vi "LVOOP Custom Probes.vi"() -> ()   [LabVIEW 2020]
doc: "This example demonstrates custom probes with LabVIEW classes.\n\nRefer to the LabVIEW Help for more information about LabVIEW object-oriented programming."
uses:
  Vehicle/Vehicle.lvclass
  Truck/Truck.lvclass
panel:
  out "truck":refnum<class "Truck.lvclass">
  out "vehicle":refnum<class "Vehicle.lvclass">
  # "See block diagram for instructions."
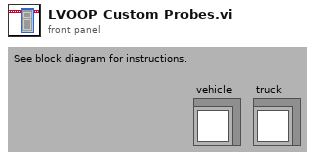
[diagram p1: front panel]
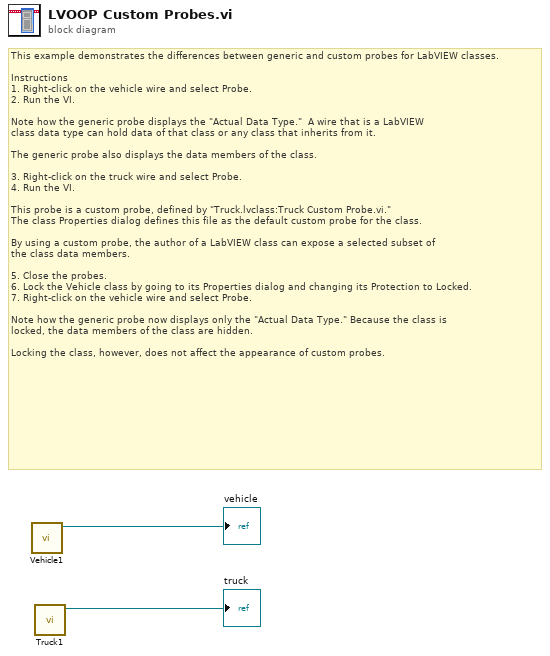
[diagram p0: block diagram]
diagram:
  # "This example demonstrates the differences between generic and custom probes for LabVIEW classes.\n\nInstructions\n1. Right-click on the vehicle wire and select Probe.\n2. Run the VI.\n\nNote how the generic probe displays the \"Actual Data Type.\"  A wire that is a LabVIEW \nclass data type can hold data of that class or any class that inherits from it.\n\nThe generic probe also displays the data members of the class.\n\n3. Right-click on the truck wire and select Probe.\n4. Run the VI.\n\nThis probe is a custom probe, defined by \"Truck.lvclass:Truck Custom Probe.vi.\"\nThe class Properties dialog defines this file as the default custom probe for the class.\n\nBy using a custom probe, the author of a LabVIEW class can expose a selected subset of\nthe class data members.\n\n5. Close the probes.\n6. Lock the Vehicle class by going to its Properties dialog and changing its Protection to Locked.\n7. Right-click on the vehicle wire and select Probe.\n\nNote how the generic probe now displays only the \"Actual Data Type.\" Because the class is\nlocked, the data members of the class are hidden.\n\nLocking the class, however, does not affect the appearance of custom probes."
  n1 = call "Vehicle1.vi"() -> ("vehicle"=→"vehicle":refnum<class "Vehicle.lvclass">)  [unwired: 11 in]
  n2 = call "Truck1.vi"() -> ("truck"=→"truck":refnum<class "Truck.lvclass">)  [unwired: 11 in]
